vi "Load Texture.vi"(6 "RGB":T1 {"B" format="%.0x"; "G" format="%.0x"; "R" format="%.0x"}, 8 "error in":errorcluster, 9 "Apply Colour Key (F)":bool, 10 "Renderer Pointer":u32 format="%.0x", 11 "File":string="c:\\temp\\hello.bmp") -> (0 "error out":errorcluster, 1 "Height":i32, 2 "Width":i32, 3 "Optimised Texture Pointer":u32 format="%.0x")   [LabVIEW 2015, in "SDL2 Utility.lvlib"]
uses:
  SDL2 Utility.lvlib
  LibSDL2 Wrapper/Controls/RGB.ctl
  LibSDL2 Wrapper/LibSDL2.lvlib
  LibSDL2_Image Wrapper/LibSDL2_Image.lvlib
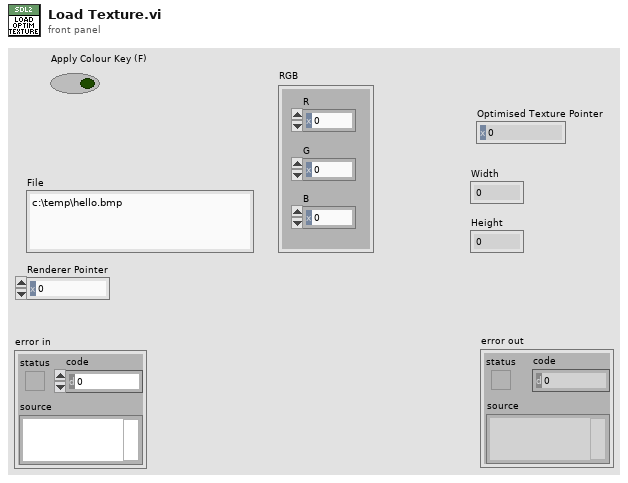
[diagram p1: front panel]
types:
  T1 = typedef "LibSDL2.lvlib/RGB.ctl" = cluster{"R":u8, "G":u8, "B":u8}
  T2 = typedef "LibSDL2.lvlib/Surface.ctl" = cluster{"Flags":u32, "Pixel Format Pointer":u32, "Width":i32, "Height":i32, "Pitch":i32, "Pixels Pointer":u32, "User Data Pointer":u32, "Locked":i32, "Lock Data Pointer":u32, "Clip Rectangle":T3, "Blitmap Pointer":u32, "Ref Count":i32}
  T3 = typedef "LibSDL2.lvlib/Rectangle.ctl" = cluster{"x":i32, "y":i32, "Width":i32, "Height":i32}
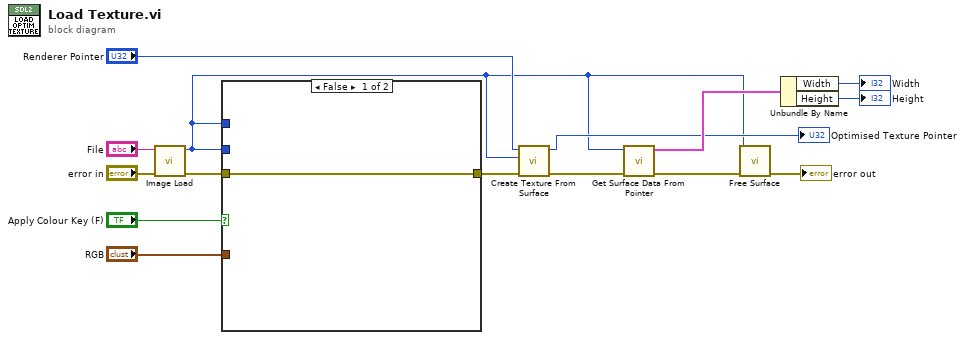
[diagram p0: block diagram]
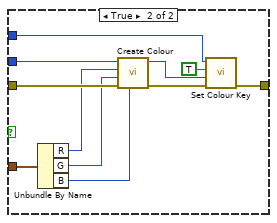
[diagram p2: hidden frame]
diagram:
  n1 = call "Image Load.vi"("error in"="error in", "File"="File") -> ("error out"=w11:errorcluster, "Surface Pointer"=w2:u32)  [unwired: 8 in]
  n2 = case shown="False" "Apply Colour Key (F)" {
    tunnel: w2 -> [_ w27]
    tunnel: w11 -> [w16 w24]
    tunnel: [w16 w25] -> w10
    tunnel: w2 -> [_ w22]
    tunnel: "RGB" -> [_ w20]
    frame False {
    }
    frame True {
      n3 = Unbundle By Name(w20) -> ("R"=w19:u8, "G"=w18:u8, "B"=w17:u8)
      n4 = call "Create Colour.vi"("B"=w17, "error in (no error)"=w24, "G"=w18, "R"=w19, "Surface Pointer"=w22) -> ("error out"=w23:errorcluster, "Colour"=w21:u32)  [unwired: 5 in]
      n5 = call "Set Colour Key.vi"("error in"=w23, "Key"=w21, "Flag"=TRUE, "Surface Pointer"=w27) -> ("error out"=w25:errorcluster)  [unwired: 6 in, 1 out]
    }
  }
  n6 = call "Create Texture From Surface.vi"("error in"=w10, "Surface Pointer"=w2, "Renderer Pointer"="Renderer Pointer") -> ("error out"=w4:errorcluster, "Texture Pointer"=→"Optimised Texture Pointer":u32)  [unwired: 7 in]
  n7 = call "Get Surface Data From Pointer.vi"("error in (no error)"=w4, "Surface Pointer"=w2) -> ("error out"=w3:errorcluster, "Surface Data"=w8:T2)  [unwired: 8 in]
  n8 = call "Free Surface.vi"("error in"=w3, "Surface Pointer"=w2) -> ("error out"=→"error out":errorcluster)  [unwired: 9 in]
  n9 = Unbundle By Name(w8) -> ("Width"=→"Width":i32, "Height"=→"Height":i32)
